vi "CRYReport Init.vi"   [LabVIEW 2013]
uses:
  CRYReport Global.vi
  CRYMainGlobal.vi
panel:
  # "Report Init."
types:
  T1 = cluster{"nCount":i16, "cFrameList":cluster{"nID":i16, "sName":string, "pVIRef":refnum<vi>, "pSPRef":refnum<vi>, "sTitle":string, "nIDObject":i16, "nIDV":i16, "nWidth":i16, "nHeight":i16, "bImgChange":bool, "sType":string, "sState":string, "sPosition":string, "sData":string}[], "sData":string}
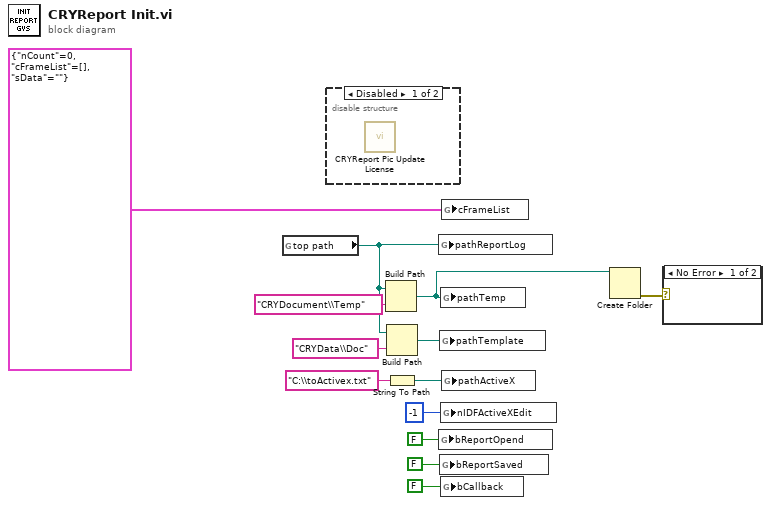
[diagram p0: block diagram]
diagram:
  n1 = global read "CRYMainGlobal.vi" "top path"() -> (w2:path)
  n2 = disable-structure shown="Disabled" {
    frame Disabled {
      n3 = call "CRYReport Pic Update License.vi"() -> ()  [unwired: 12 in]
    }
    frame Enabled {
    }
  }
  n4 = Build Path(base path=w2, name or relative path="CRYDocument\\Temp") -> (appended path=w4:path)
  n5 = Build Path(base path=w2, name or relative path="CRYData\\Doc") -> (appended path=w1:path)
  n6 = String To Path(string="C:\\toActivex.txt" ("name or relative path")) -> (path=w10:path)
  n7 = global write "CRYReport Global.vi" "pathReportLog"(w2) -> ()
  n8 = global write "CRYReport Global.vi" "bReportOpend"(FALSE ("bPreportOpend")) -> ()
  n9 = global write "CRYReport Global.vi" "pathTemplate"(w1) -> ()
  n10 = global write "CRYReport Global.vi" "bReportSaved"(FALSE ("bPreportOpend")) -> ()
  n11 = global write "CRYReport Global.vi" "pathTemp"(w4) -> ()
  n12 = global write "CRYReport Global.vi" "nIDFActiveXEdit"(i16 -1 ("nIDFActiveXEdit")) -> ()
  n13 = global write "CRYReport Global.vi" "bCallback"(FALSE ("bPreportOpend")) -> ()
  n14 = global write "CRYReport Global.vi" "cFrameList"(T1 {"nCount"=0, "cFrameList"=[], "sData"=""} ("cFrameList")) -> ()
  n15 = global write "CRYReport Global.vi" "pathActiveX"(w10) -> ()
  n16 = Create Folder(path (use dialog)=w4) -> (error out=w5:errorcluster)  [unwired: 2 in, 2 out]
  n17 = case shown="No Error" w5 {
    frame No Error {
    }
    frame Error {
    }
  }
